vi "Peak at Message.vi"(0 "Listening Queue":refnum<queue>, 5 "timeout in ms (-1)":i32=-1, 11 "error in (no error)":errorcluster) -> (2 "Source":string, 3 "Destination":string, 4 "queue out":refnum<queue>, 6 "Command":string, 10 "Data":variant, 14 "Time Stamp":timestamp, 15 "error out":errorcluster)   [LabVIEW 2020, in "Dynamic Reentrant.lvlib"]
uses:
  Dynamic Reentrant.lvlib
  Type Defs/Message.ctl
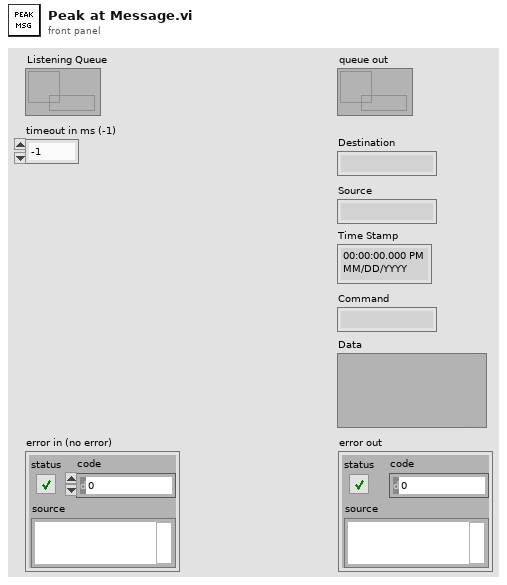
[diagram p1: front panel]
types:
  T1 = typedef "Dynamic Reentrant.lvlib/Message.ctl" = cluster{"Source":string, "Destination":string, "Time Stamp":timestamp, "Command":string, "Data":variant}
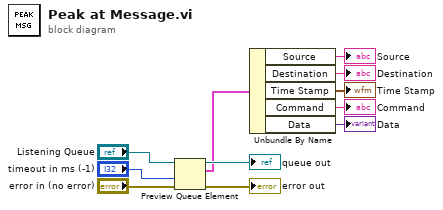
[diagram p0: block diagram]
diagram:
  n1 = Preview Queue Element(queue="Listening Queue", timeout in ms (-1)="timeout in ms (-1)", error in (no error)="error in (no error)") -> (queue out=→"queue out":refnum<queue>, element=w6:T1, error out=→"error out":errorcluster)  [unwired: 1 out]
  n2 = Unbundle By Name(w6) -> ("Source"=→"Source":string, "Destination"=→"Destination":string, "Time Stamp"=→"Time Stamp":timestamp, "Command"=→"Command":string, "Data"=→"Data":variant)
